vi "Remote PC - Server.vi"() -> ()   [LabVIEW 2012]
panel:
  out "Message":string
  # "WLAN Remote Sever Running..."
  # "WLAN Remote Sever Running..."
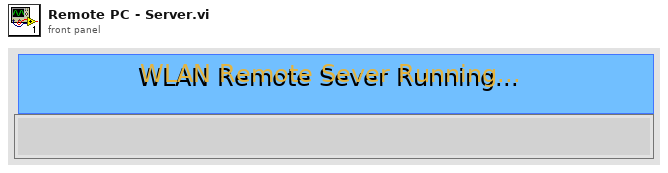
[diagram p1: front panel]
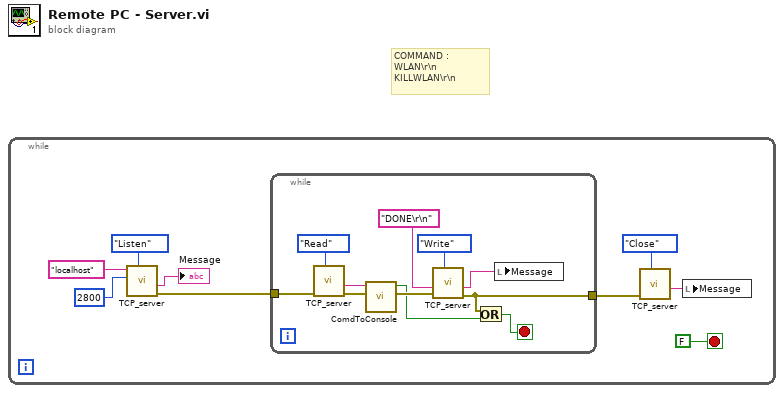
[diagram p0: block diagram]
diagram:
  # "COMMAND :        \nWLAN\\r\\n\nKILLWLAN\\r\\n"
  n1 = while {
    stop <- FALSE stop-if-true
    n2 = call "TCP_server.vi"("Flow Control"=enum16{"Listen", "Read", "Write", "Close"}."Listen" ("TCP ctrl"), "Local Server Port"=u16 2800 ("port"), "service name"="localhost") -> ("error out"=w5:errorcluster, "Message"=→"Message":string)  [unwired: 7 in]
    n3 = while {
      tunnel: w5 -> [w19]
      tunnel: [w13] -> w4
      stop <- w11 stop-if-true
      n4 = call "TCP_server.vi"("Flow Control"=enum16{"Listen", "Read", "Write", "Close"}."Read" ("TCP ctrl"), "error in"=w19) -> ("error out"=w18:errorcluster, "Message"=w17:string)  [unwired: 8 in]
      n5 = call "ComdToConsole.vi"("error in"=w18, "command"=w17) -> ("error out"=w14:errorcluster, "Disconnect?"=w12:bool)  [unwired: 5 in]
      n6 = call "TCP_server.vi"("Flow Control"=enum16{"Listen", "Read", "Write", "Close"}."Write" ("TCP ctrl"), "error in"=w14, "Send Message"="DONE\r\n") -> ("error out"=w13:errorcluster, "Message"=w10:string)  [unwired: 7 in]
      n7 = Or(x=w13, y=w12) -> (x .or. y?=w11:bool)
      n8 = local write "Message"(w10) -> ()
    }
    n9 = call "TCP_server.vi"("Flow Control"=enum16{"Listen", "Read", "Write", "Close"}."Close" ("TCP ctrl"), "error in"=w4) -> ("Message"=w2:string)  [unwired: 8 in, 1 out]
    n10 = local write "Message"(w2) -> ()
  }
